vi "qFRH.vi"(0 "System no.":i32=1 min=1 max=4 step=1, 5 "error in":errorcluster) -> (14 "FRR? help string":string, 15 "FRR? help string parsed":T1(array[cluster]), 16 "ResultID Out":i32[](array[numeric]), 17 "Meaning Out":string[](array[string]), 18 "Value Unit Out":string[](array[string]), 19 "error out":errorcluster)   [LabVIEW 2026]
doc: "The command returns an ASCII help string with available query options (\"result IDs\") for the FRR? command. \n\nC-887, E-712, E-727.AS:"
panel:
  # "Get  help for FRR? command."
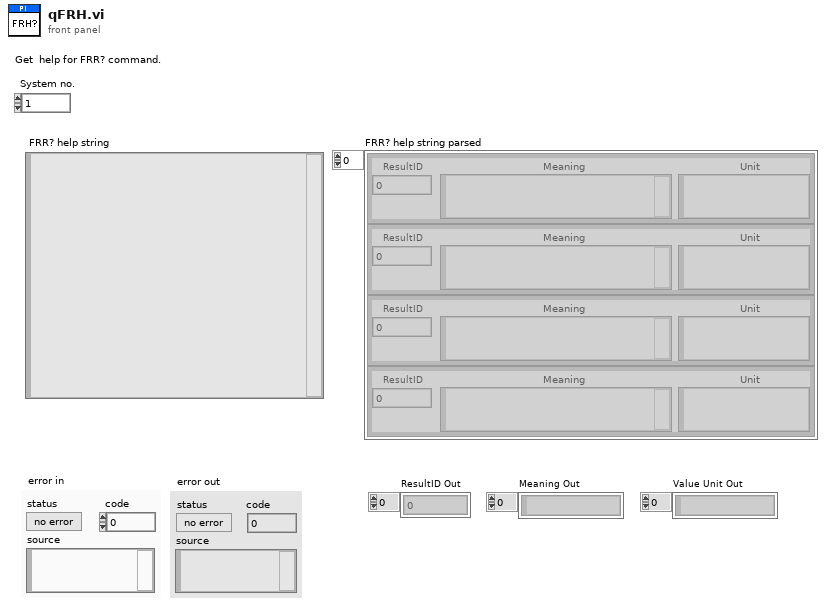
[diagram p1: front panel]
types:
  T1 = cluster{"ResultID":i32, "Meaning":string, "Unit":string}[]
  T2 = cluster{"ID":i32, "String 1":string, "String 2":string}[]
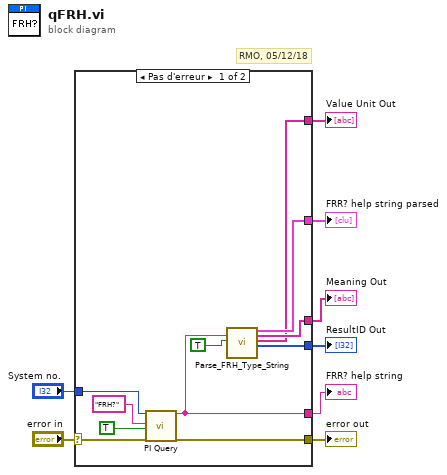
[diagram p0: block diagram]
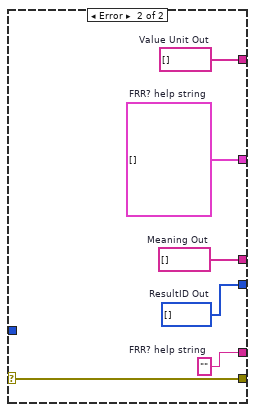
[diagram p2: hidden frame]
diagram:
  # "RMO, 05/12/18"
  n1 = case shown="Pas d'erreur" "error in" {
    selector: "error in" -> [w11 w25]
    tunnel: [w16 w24] -> w8
    tunnel: [w15 w23] -> w7
    tunnel: [w14 w21] -> w6
    tunnel: [w13 w22] -> w5
    tunnel: [w12 w25] -> w4
    tunnel: "System no." -> [w10 _]
    tunnel: [w9 w20] -> w1
    frame No Error {
      n2 = call "PI Query.vi"("System no."=w10, "String to send"="FRH?" ("String to Send"), "Attach termination char.?"=TRUE ("Attach Linefeed?"), "error in"=w11) -> ("String read"=w9:string, "error out"=w12:errorcluster)  [unwired: 3 in, 11 out]
      n3 = call "Parse_FRH_Type_String.vi"("String In"=w9, "All IDs?"=TRUE) -> ("Parsed Cluster Out"=w16:T2, "String 1 Out"=w15:string[], "String 2 Out"=w14:string[], "IDs Out"=w13:i32[])  [unwired: 1 in, 13 out]
    }
    frame Error {
      w21 = string[] []  # Value Unit Out
      w22 = i32[] []  # ResultID Out
      w23 = string[] []  # Meaning Out
      w24 = T2 []  # FRR? help string
      w20 = ""  # FRR? help string
    }
  }
  "error out" <- w4
  "FRR? help string parsed" <- w8
  "ResultID Out" <- w5
  "Meaning Out" <- w7
  "Value Unit Out" <- w6
  "FRR? help string" <- w1
